vi "OLD 2D Motion Profiling.vi"() -> ()   [LabVIEW 2016]
uses:
  <vilib>/gmath/NI_Gmath.lvlib
  <vilib>/Analysis/NI_AALPro.lvlib
panel:
  out "XY Graph":cluster{dbl[], "dX/dt":dbl[]}[](graph)
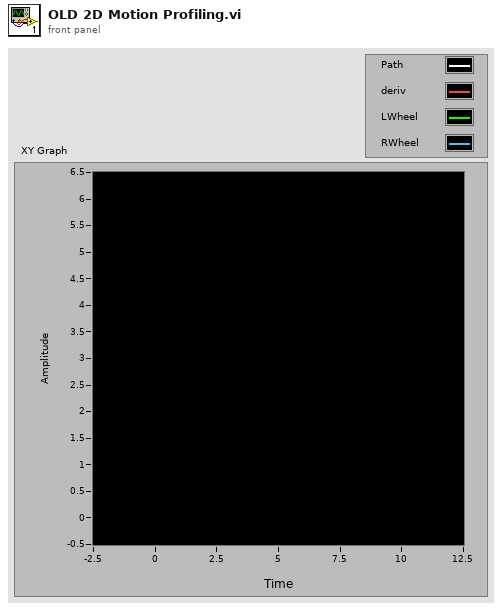
[diagram p1: front panel]
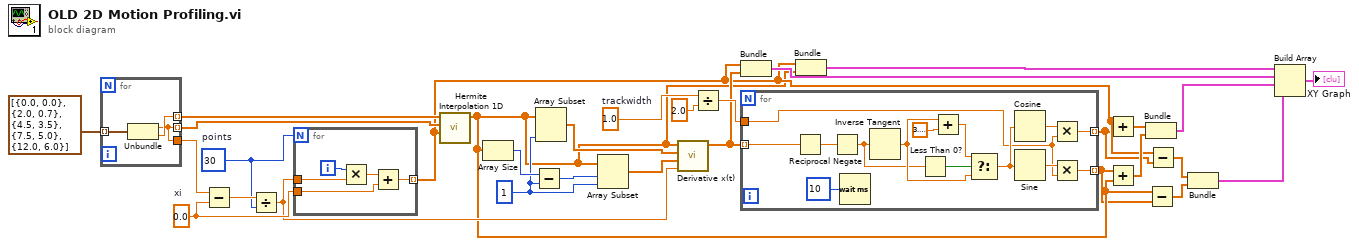
[diagram p0: block diagram]
diagram:
  w16 = 1.0  # trackwidth
  w18 = 1 ("length")
  w26 = 30  # points
  w25 = 0.0  # xi
  n1 = for {
    tunnel: cluster{"X":dbl, "Y":dbl}[] [{"X"=0.0, "Y"=0.0}, {"X"=2.0, "Y"=0.7}, {"X"=4.5, "Y"=3.5}, {"X"=7.5, "Y"=5.0}, {"X"=12.0, "Y"=6.0}] ("x/y") -> [w33] mode=indexing
    tunnel: [w31] -> w30 mode=indexing
    tunnel: [w32] -> w29 mode=indexing
    tunnel: [w31] -> w17
    n2 = Unbundle(w33) -> ("X"=w31:dbl, "Y"=w32:dbl)
  }
  n3 = Subtract(x=w17, y=w25) -> (x-y=w27:dbl)
  n4 = Divide(x=w27, y=w26) -> (x/y=w24:dbl)
  n5 = for {
    N: w26 -> [_]
    tunnel: [w34] -> w7 mode=indexing
    tunnel: w24 -> [w37]
    tunnel: w25 -> [w35]
    i -> [w38]
    n6 = Multiply(x=w38, y=w37) -> (x*y=w36:dbl)
    n7 = Add(x=w36, y=w35) -> (x+y=w34:dbl)
  }
  n8 = call <vilib>:"Hermite Interpolation 1D.vi"("xi"=w7, "X"=w30, "Y"=w29) -> ("yi"=w5:dbl[])  [unwired: 6 in, 2 out]
  n9 = Array Size(array=w5) -> (size(s)=w21:i32)
  n10 = Subtract(x=w21, y=w18) -> (x-y=w20:i32)
  n11 = Array Subset(array=w5, length=w18) -> (w22:dbl[])  [unwired: 1 in]
  n12 = Array Subset(array=w5, index=w20, length=w18) -> (w19:dbl[])
  n13 = call <vilib>:"Derivative x(t).vi"("dt"=w24, "Final Condition"=w19, "Initial Condition"=w22, "X"=w5) -> ("dX/dt"=w13:dbl[])  [unwired: 6 in, 1 out]
  n14 = Divide(x=w16, y=2.0) -> (x/y=w14:dbl)
  n15 = Bundle(w7, "dX/dt"=w13) -> (w23:cluster{dbl[], "dX/dt":dbl[]})  [unwired: 1 in]
  n16 = for {
    tunnel: w13 -> [w52] mode=indexing
    tunnel: w14 -> [w42]
    tunnel: [w41] -> w6 mode=indexing
    tunnel: [w40] -> w4 mode=indexing
    n17 = Reciprocal(x=w52) -> (1/x=w51:dbl)
    n18 = Negate(x=w51) -> (-x=w43:dbl)
    n19 = Wait (ms)(milliseconds to wait=u32 10) -> ()  [unwired: 1 out]
    n20 = Inverse Tangent(1:w43) -> (0:w45:dbl)
    n21 = Less Than 0?(x=w43) -> (x < 0?=w44:bool)
    n22 = Add(x=w45, y=3.141592653589793) -> (x+y=w47:dbl)
    n23 = Select(t=w47, s=w44, f=w45) -> (s? t:f=w48:dbl)
    n24 = Cosine(x=w48) -> (cos(x)=w49:dbl)
    n25 = Sine(x=w48) -> (sin(x)=w50:dbl)
    n26 = Multiply(x=w49, y=w42) -> (x*y=w41:dbl)
    n27 = Multiply(x=w50, y=w42) -> (x*y=w40:dbl)
  }
  n28 = Bundle(w7, "yi"=w5) -> (w28:cluster{dbl[], "yi":dbl[]})  [unwired: 1 in]
  n29 = Add(x=w7, y=w6) -> (x+y=w12:dbl[])
  n30 = Add(x=w4, y=w5) -> (x+y=w11:dbl[])
  n31 = Bundle(w12, w11) -> (w10:cluster{dbl[], dbl[]})  [unwired: 1 in]
  n32 = Subtract(x=w5, y=w4) -> (x-y=w2:dbl[])
  n33 = Subtract(x=w7, y=w6) -> (x-y=w3:dbl[])
  n34 = Bundle(w3, w2) -> (w1:cluster{dbl[], dbl[]})  [unwired: 1 in]
  n35 = Build Array(w28, w23, w10, w1) -> (→"XY Graph":cluster{dbl[], "dX/dt":dbl[]}[])
